vi "Piezo wiggle - high level.vi"() -> ()   [LabVIEW 2017]
uses:
  Global wiggle variables.vi
panel:
  in  "ON/OFF":bool
  in  "Amplitude":dbl=37.5 min=0.0 max=75.0
  in  "Frequency (Hz)":dbl=1.0
  in  "stop main VI":bool
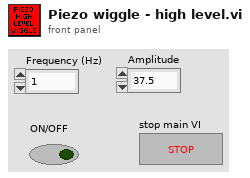
[diagram p1: front panel]
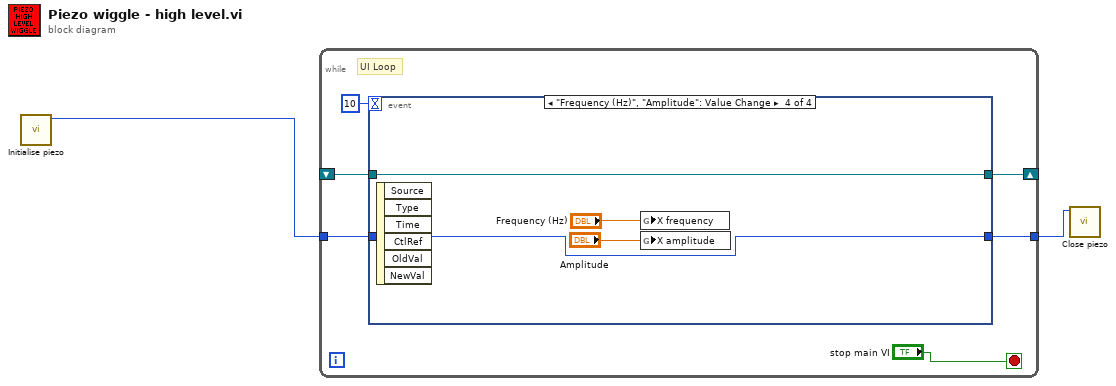
[diagram p0: block diagram]
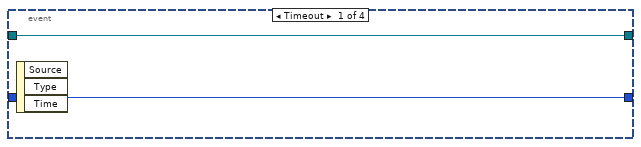
[diagram p2: hidden frame]
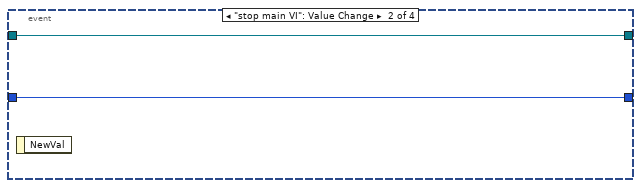
[diagram p3: hidden frame]
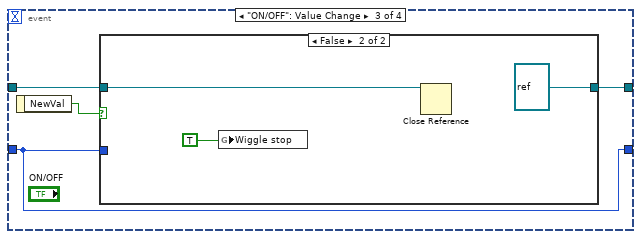
[diagram p4: hidden frame]
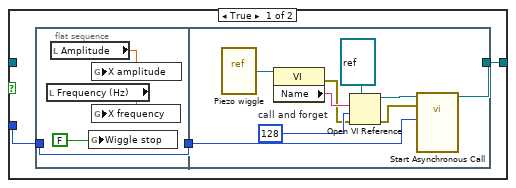
[diagram p5: hidden frame]
diagram:
  n1 = call "Initialise piezo.vi"() -> ("Piezo handle"=w2:i32)  [unwired: 10 in, 1 out]
  n2 = while {
    tunnel: w2 -> [w8]
    shift-right: [w7] -> _
    shift-left: _ -> [w6]
    tunnel: [w3] -> w1
    stop <- "stop main VI" stop-if-true
    # "UI Loop"
    n3 = event shown="[3] \"Frequency (Hz)\", \"Amplitude\": Value Change" {
      selector: _ -> [_ _ _ _]
      dyn-events: _ -> [_ _ _ _]
      timeout: 10 -> [_ _ _ _]
      tunnel: w8 -> [w9 w11 w16 w36]
      tunnel: [w10 w12 w15 w37] -> w7
      tunnel: w6 -> [w10 w12 w13 w37]
      tunnel: [w9 w11 w16 w36] -> w3
      event Timeout {
        n4 = event-data() -> ()  [unwired: 1 in, 3 out]
      }
      event "stop main VI": Value Change {
        n5 = event-data() -> ()  [unwired: 1 in, 1 out]
      }
      event "ON/OFF": Value Change {
        n6 = event-data() -> ("NewVal"=w14:bool)  [unwired: 1 in]
        n7 = case shown="False" w14 {
          tunnel: w16 -> [w19 _]
          tunnel: [w18 refnum<vi> refnum ("type specifier VI Refnum (for type only)")] -> w15
          tunnel: w13 -> [_ w33]
          frame True {
            n8 = flat-sequence {
              tunnel: w19 -> [w23]
              tunnel: [w23] -> w17
              tunnel: [w24] -> w18
              tunnel: w17 -> [w25]
              frame #0 {
                n9 = local read "Frequency (Hz)"() -> (w20:dbl)
                n10 = local read "Amplitude"() -> (w21:dbl)
                n11 = global write "Global wiggle variables.vi" "Wiggle stop"(FALSE) -> ()
                n12 = global write "Global wiggle variables.vi" "X amplitude"(w21) -> ()
                n13 = global write "Global wiggle variables.vi" "X frequency"(w20) -> ()
              }
              frame #1 {
                w30 = 128  # call and forget
                n14 = vi-ref "Piezo wiggle.vi"() -> (w32:refnum<vi>)
                n15 = property class="VI"(reference=w32) -> (error out=w29:errorcluster, "Name"=w31:string)  [unwired: 1 in, 1 out]
                n16 = Open VI Reference(type specifier VI Refnum (for type only)=refnum<vi> refnum, vi path=w31, options=w30, error in (no error)=w29) -> (vi reference=w27:refnum<vi>, error out=w26:errorcluster)  [unwired: 2 in]
                n17 = call-by-ref "Start Asynchronous Call"(reference=w27, error in=w26, "Piezo handle in"=w25) -> (reference out=w24:refnum<vi>)  [unwired: 7 in, 3 out]
              }
            }
          }
          frame False {
            n18 = global write "Global wiggle variables.vi" "Wiggle stop"(TRUE) -> ()
            n19 = Close Reference(reference=w33) -> ()  [unwired: 1 in, 1 out]
          }
        }
      }
      event "Frequency (Hz)", "Amplitude": Value Change {
        n20 = event-data() -> ()  [unwired: 1 in, 6 out]
        n21 = global write "Global wiggle variables.vi" "X frequency"("Frequency (Hz)") -> ()
        n22 = global write "Global wiggle variables.vi" "X amplitude"("Amplitude") -> ()
      }
    }
  }
  n23 = call "Close piezo.vi"("Piezo handle"=w1) -> ()  [unwired: 10 in, 1 out]
